vi "Add message line.vi"(8 "error in (no error)":errorcluster, 10 "Message in":string, 11 "Chat in":refnum<class "Chat.lvclass">) -> (0 "error out":errorcluster, 3 "Chat out":refnum<class "Chat.lvclass">)   [LabVIEW 2012, in "Chat.lvclass"]
uses:
  Chat.lvclass
  Chat.lvclass/Chat.ctl
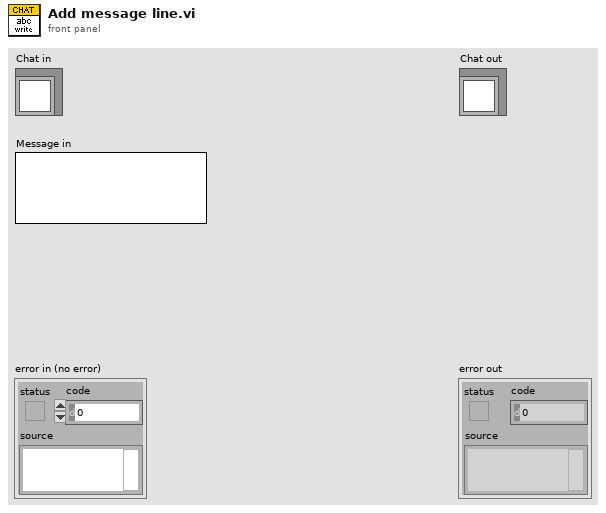
[diagram p1: front panel]
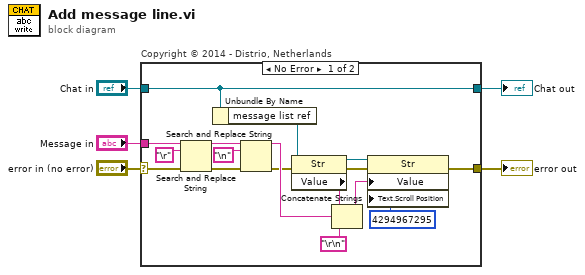
[diagram p0: block diagram]
diagram:
  n1 = case "Copyright © 2014 - Distrio, Netherlands" shown="No Error" "error in (no error)" {
    selector: "error in (no error)" -> [w8 w24]
    tunnel: [w20 w24] -> w4
    tunnel: [w22 w23] -> w2
    tunnel: "Chat in" -> [w22 w23]
    tunnel: "Message in" -> [w10 _]
    frame No Error {
      n2 = Search and Replace String(input string=w10, search string="\r", error in=w8) -> (result string=w9:string, error out=w7:errorcluster)  [unwired: 5 in, 2 out]
      n3 = Unbundle By Name(w22) -> ("message list ref"=w21:refnum<vi>)
      n4 = Search and Replace String(input string=w9, search string="\n", error in=w7) -> (result string=w14:string, error out=w13:errorcluster)  [unwired: 5 in, 2 out]
      n5 = property class="Str"(reference=w21, error in=w13) -> (reference out=w17:refnum<vi>, error out=w19:errorcluster, "Value"=w18:string)
      n6 = Concatenate Strings(w18, w14, "\r\n") -> (w16:string)
      n7 = property class="Str"(reference=w17, error in=w19, "Value"=w16, "Text.Scroll Position"=u32 4294967295) -> (error out=w20:errorcluster)  [unwired: 1 out]
    }
    frame Error {
    }
  }
  "error out" <- w4
  "Chat out" <- w2
